vi "relative_link.vi"   [LabVIEW 2021]
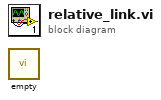
[diagram p0: block diagram]
diagram:
  n1 = call "empty.vi"() -> ()  [unwired: 12 in]
